vi "Migrate Process Config.vi"(8 "error in (no error)":errorcluster, 10 "Old Process Config":path, 11 "App Data Directory":path) -> (0 "error out":errorcluster)   [LabVIEW 2020, in "MacroAssert.lvlib"]
doc: "Migrates any old macros from the old location to the new location."
uses:
  MacroAssert.lvlib
  <vilib>/Utility/config.llb/NI_LVConfig.lvlib
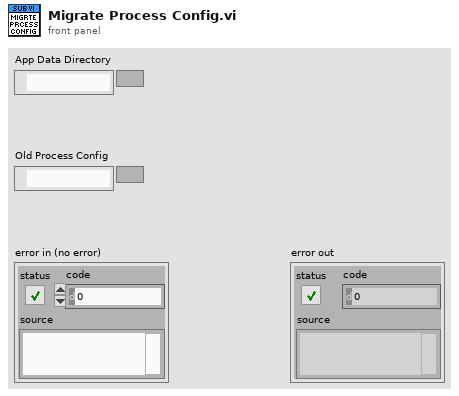
[diagram p1: front panel]
types:
  T1 = typedef "NI_LVConfig.lvlib/Config Data RefNum.ctl" = refnum<k1>
  T2 = typedef "MacroAssert.lvlib/Macro Cluster V3.ctl" = cluster{"Config":T3, "Steps":T4[]}
  T3 = typedef "MacroAssert.lvlib/Macro Config V3.ctl" = cluster{"Schema Version":string, "Activation Type":enum32{"Hotkey", "Automatic"}, "N":i32, "Description":string, "Resolutions":cluster{"Width":i16, "Height":i16}[], "Date Created":timestamp, "Date Updated":timestamp}
  T4 = typedef "MacroAssert.lvlib/Step V3.ctl" = cluster{"Type":T5, "X":i32, "Y":i32, "Delay":i32, "Key":u8, "Repeat":i32, "RClick?":bool, "App/Window Name":string, "Notes":string}
  T5 = typedef "MacroAssert.lvlib/Step Type V3.ctl" = enum16{"Mouse Move", "Mouse Click", "Key Press", "Wait", "Mouse Down", "Mouse Up", "Key Down", "Key Up", "Run Application", "Maximize Window", "Restore Window", "Minimize Window", "Close Window", "Bring Window to Front", "Send Window to Back"}
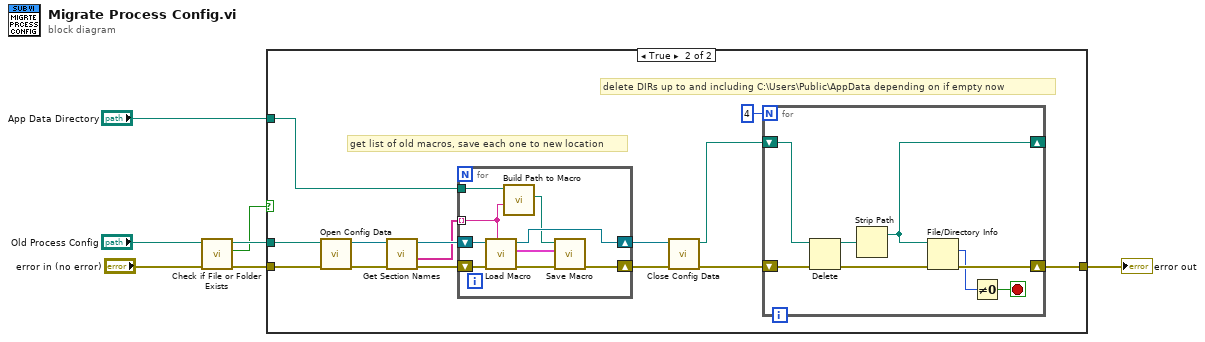
[diagram p0: block diagram]
diagram:
  n1 = call <vilib>:"Check if File or Folder Exists.vi"("error in (no error)"="error in (no error)", "path"="Old Process Config") -> ("error out"=w5:errorcluster, "file or folder exists?"=w2:bool, "dup path"=w6:path)  [unwired: 7 in]
  n2 = case shown="True" w2 {
    tunnel: w6 -> [_ w19]
    tunnel: w5 -> [w8 w20]
    tunnel: "App Data Directory" -> [_ w13]
    tunnel: [w8 w22] -> w3
    frame False {
    }
    frame True {
      # "delete DIRs up to and including C:\\Users\\Public\\AppData depending on if empty now"
      # "get list of old macros, save each one to new location"
      n3 = call <vilib>:"Open Config Data.vi"("error in (no error)"=w20, "configuration file path"=w19) -> ("error out"=w18:errorcluster, "refnum"=w17:T1)  [unwired: 7 in, 1 out]
      n4 = call <vilib>:"Get Section Names.vi"("error in (no error)"=w18, "refnum"=w17) -> ("error out"=w16:errorcluster, "section names"=w14:string[], "refnum out"=w15:T1)  [unwired: 7 in]
      n5 = for {
        shift-right: [w31] -> w12
        shift-left: w16 -> [w30]
        shift-right: [w27] -> w11
        shift-left: w15 -> [w29]
        tunnel: w14 -> [w24] mode=indexing
        tunnel: w13 -> [w25]
        n6 = call "Load Macro.vi"("Macro Name"=w24, "error in (no error)"=w30, "refnum"=w29) -> ("error out"=w28:errorcluster, "Macro"=w26:T2, "refnum out"=w27:T1)  [unwired: 6 in]
        n7 = call "Build Path to Macro.vi"("Macro Name"=w24, "App Data Dir"=w25) -> ("Macro File Path"=w23:path)  [unwired: 9 in]
        n8 = call "Save Macro.vi"("error in (no error)"=w28, "Macro Cluster"=w26, "File Path"=w23) -> ("error out"=w31:errorcluster)  [unwired: 8 in]
      }
      n9 = call <vilib>:"Close Config Data.vi"("error in (no error)"=w12, "refnum"=w11) -> ("error out"=w10:errorcluster, "file path"=w9:path)  [unwired: 8 in]
      n10 = for {
        N: 4 -> [_]
        shift-right: [w32] -> _
        shift-left: w9 -> [w38]
        shift-right: [w35] -> w22
        shift-left: w10 -> [w39]
        stop <- w33 stop-if-true
        n11 = Delete(path (use dialog)=w38, error in=w39) -> (deleted path=w37:path, error out=w36:errorcluster)  [unwired: 3 in, 1 out]
        n12 = Strip Path(path=w37) -> (stripped path=w32:path)  [unwired: 1 out]
        n13 = File/Directory Info(path=w32, error in=w36) -> (size=w34:i64, error out=w35:errorcluster)  [unwired: 5 out]
        n14 = Not Equal To 0?(x=w34) -> (x != 0?=w33:bool)
      }
    }
  }
  "error out" <- w3
